vi "eliminarobjetobase.vi"(9 "Nombre objeto a eliminar":string) -> ()   [LabVIEW 2020]
doc: "Este VI elimina el objeto indicado en \"Nombre objeto a eliminar\" en la base de datos especificada en la variable global."
uses:
  Global_archivobasedatos.vi
  <vilib>/addons/database/Connection.llb/DB Tools Open Connec (Path).vi
  <vilib>/addons/database/Connection.llb/Conn Execute.vi
  <vilib>/addons/database/Recordset.llb/Rec Destroy - Connection.vi
  <vilib>/addons/database/NI_Database_API.lvlib
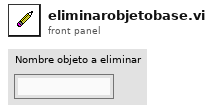
[diagram p1: front panel]
types:
  T1 = typedef "NI_Database_API.lvlib/Conn ObjectReference.ctl" = refnum<k1>
  T2 = typedef "NI_Database_API.lvlib/Rec ObjectReference.ctl" = refnum<k1>
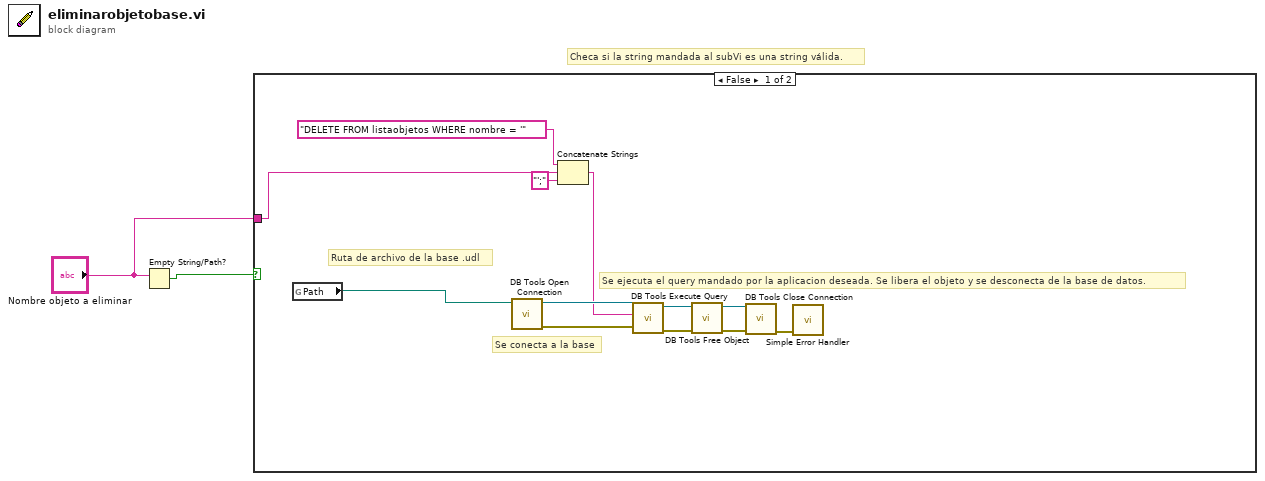
[diagram p0: block diagram]
diagram:
  # "Checa si la string mandada al subVi es una string válida."
  n1 = Empty String/Path?(string/path="Nombre objeto a eliminar") -> (empty?=w2:bool)
  n2 = case shown="False" w2 {
    tunnel: "Nombre objeto a eliminar" -> [w5 _]
    frame False {
      # "Se ejecuta el query mandado por la aplicacion deseada. Se libera el objeto y se desconecta de la base de datos."
      # "Se conecta a la base"
      # "Ruta de archivo de la base .udl"
      n3 = global read "Global_archivobasedatos.vi" "Path"() -> (w7:path)
      n4 = call-poly <vilib>:"DB Tools Open Connection.vi"("connection information"=w7) -> ("error out"=w11:errorcluster, "connection reference"=w10:T1)  [unwired: 7 in]
      n5 = Concatenate Strings("DELETE FROM listaobjetos WHERE nombre = '", w5, "';" ("string")) -> (w3:string)
      n6 = call-poly <vilib>:"DB Tools Execute Query.vi"("error in (no error)"=w11, "SQL query"=w3, "connection reference"=w10) -> ("error out"=w8:errorcluster, "recordset reference"=w9:T2)  [unwired: 5 in]
      n7 = call-poly <vilib>:"DB Tools Free Object.vi"("error in (no error)"=w8, "recordset reference"=w9) -> ("error out"=w13:errorcluster, "connection reference"=w14:T1)  [unwired: 8 in]
      n8 = call <vilib>:"DB Tools Close Connection.vi"("error in (no error)"=w13, "connection reference"=w14) -> ("error out"=w12:errorcluster)  [unwired: 5 in]
      n9 = call <vilib>:"Simple Error Handler.vi"("error in (no error)"=w12) -> ()  [unwired: 4 in, 5 out]
    }
    frame True {
    }
  }
